vi "test Sort Array of Clusters Natural String Sort.vi"(8 "error in (no error)":errorcluster, 11 "TestCase in":refnum<class "UI Common Unit Tests.lvclass">) -> (0 "error out":errorcluster, 3 "TestCase out":refnum<class "UI Common Unit Tests.lvclass">)   [LabVIEW 2017, in "UI Common Unit Tests.lvclass"]
uses:
  UI Common Unit Tests.lvclass
  Array Row.ctl
  63dc8703-c824-4b80-a085-58f57073aca5.vi
  d8dc5a30-59fd-40f1-b092-92b0634dc405.vi
  c62d43f3-ccf2-448e-89d3-d67a32af4b30.vi
  0d07b81e-88f3-4258-8836-385d3b76f707.vi
  63dc8703-c824-4b80-a085-58f57073aca5.vi/7dda6a87-888e-4219-9294-afb2d8f7f202.vi
  63dc8703-c824-4b80-a085-58f57073aca5.vi/7a811afe-08d6-4889-9a6b-707c54def933.vi
  d8dc5a30-59fd-40f1-b092-92b0634dc405.vi/55d2f0e8-b25a-4c34-86b0-45c4342d676d.vi
  d8dc5a30-59fd-40f1-b092-92b0634dc405.vi/529c5265-cbd4-4584-81ba-3b6ee758e69e.vi
  c62d43f3-ccf2-448e-89d3-d67a32af4b30.vi/6e754a95-77fb-4ec3-a969-ba8b3d19ed54.vi
  c62d43f3-ccf2-448e-89d3-d67a32af4b30.vi/98e32075-a747-4c62-ac3b-b709402c5c03.vi
  0d07b81e-88f3-4258-8836-385d3b76f707.vi/cc1b897a-72e7-4acf-8e52-5fbb4102f40d.vi
  0d07b81e-88f3-4258-8836-385d3b76f707.vi/2126984c-6580-428d-86be-ed2c8ec06a10.vi
  Natural String Merge Sort.vi
  <vilib>/addons/_JKI Toolkits/VI Tester/TestCase.llb/TestCase.lvclass
  C:/Program Files (x86)/National Instruments/LabVIEW 2017/vi.lib/addons/_JKI Toolkits/VI Tester/TestCase.llb/TestCase.lvclass
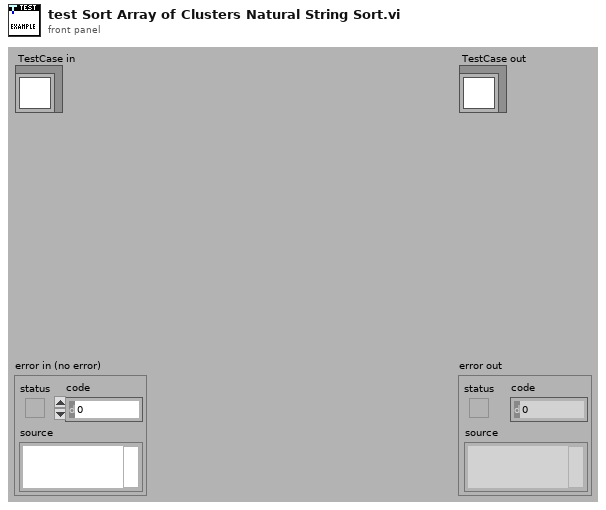
[diagram p1: front panel]
types:
  T1 = typedef "UI Common Unit Tests.lvclass/Array Row.ctl" = cluster{"String":string, "Numeric":dbl}
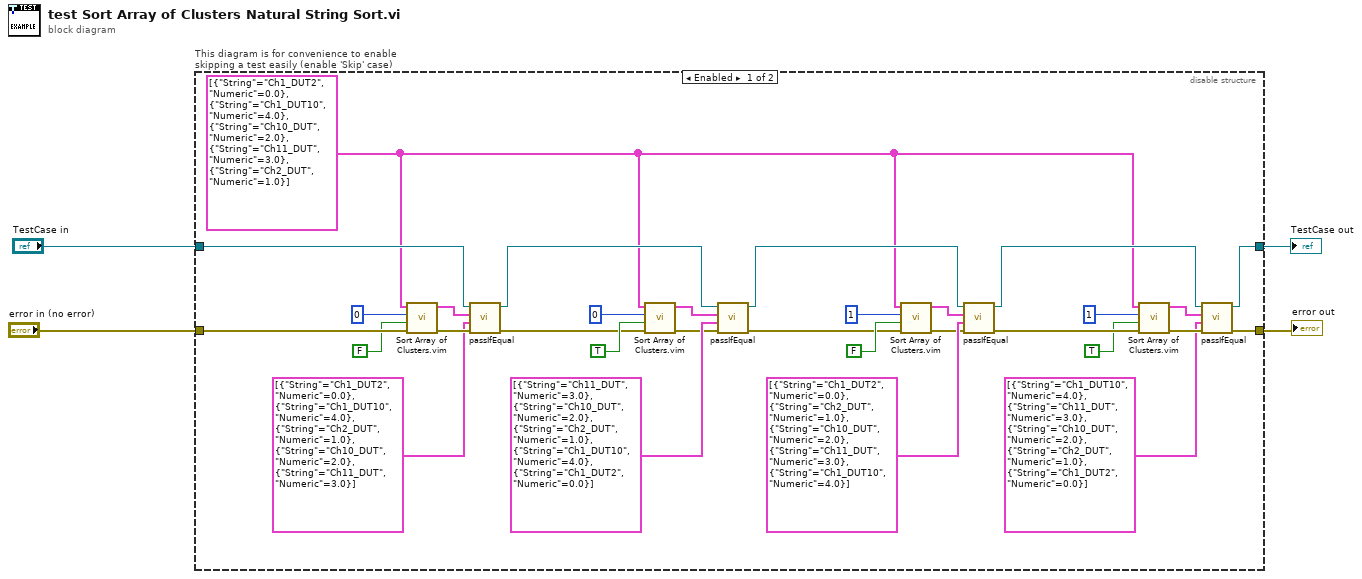
[diagram p0: block diagram]
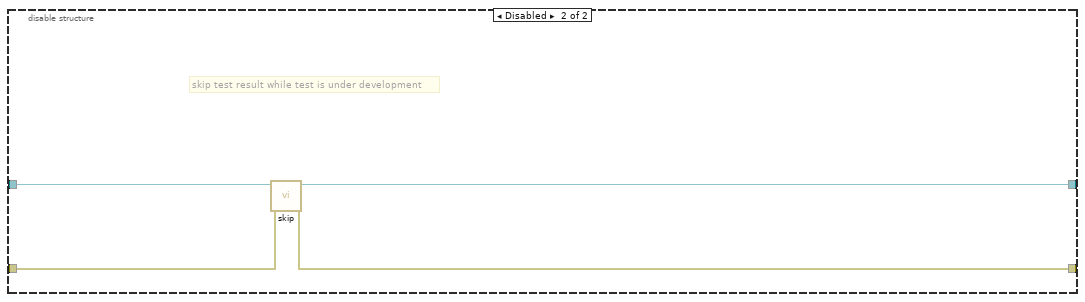
[diagram p2: hidden frame]
diagram:
  n1 = disable-structure "This diagram is for convenience to enable skipping a test easily (enable 'Skip' case)" shown="Enabled" {
    disable-tunnel: "TestCase in" -> [w31 w39]
    disable-tunnel: [w10 w37] -> w1
    disable-tunnel: [w6 w38] -> w3
    disable-tunnel: "error in (no error)" -> [w35 w36]
    frame Enabled {
      w5 = T1[] [{"String"="Ch1_DUT2", "Numeric"=0.0}, {"String"="Ch1_DUT10", "Numeric"=4.0}, {"String"="Ch10_DUT", "Numeric"=2.0}, {"String"="Ch11_DUT", "Numeric"=3.0}, {"String"="Ch2_DUT", "Numeric"=1.0}] ("Value")
      n2 = call "Sort Array of Clusters.vim"("error in (no error)"=w35, "Descending"=FALSE, "index"=u32 0, "Array"=w5) -> ("error out"=w32:errorcluster, "Sorted Array"=w30:T1[])  [unwired: 6 in]
      n3 = call-dynamic "passIfEqual.vi"("error in (no error)"=w32, "y"=T1[] [{"String"="Ch1_DUT2", "Numeric"=0.0}, {"String"="Ch1_DUT10", "Numeric"=4.0}, {"String"="Ch2_DUT", "Numeric"=1.0}, {"String"="Ch10_DUT", "Numeric"=2.0}, {"String"="Ch11_DUT", "Numeric"=3.0}] ("Value"), "x"=w30, "TestCase in"=w31) -> ("error out"=w23:errorcluster, "TestCase out"=w22:refnum<class "UI Common Unit Tests.lvclass">)  [unwired: 6 in]
      n4 = call "Sort Array of Clusters.vim"("error in (no error)"=w23, "Descending"=TRUE, "index"=u32 0, "Array"=w5) -> ("error out"=w26:errorcluster, "Sorted Array"=w27:T1[])  [unwired: 6 in]
      n5 = call-dynamic "passIfEqual.vi"("error in (no error)"=w26, "y"=T1[] [{"String"="Ch11_DUT", "Numeric"=3.0}, {"String"="Ch10_DUT", "Numeric"=2.0}, {"String"="Ch2_DUT", "Numeric"=1.0}, {"String"="Ch1_DUT10", "Numeric"=4.0}, {"String"="Ch1_DUT2", "Numeric"=0.0}] ("Value"), "x"=w27, "TestCase in"=w22) -> ("error out"=w7:errorcluster, "TestCase out"=w8:refnum<class "UI Common Unit Tests.lvclass">)  [unwired: 6 in]
      n6 = call "Sort Array of Clusters.vim"("error in (no error)"=w7, "Descending"=FALSE, "index"=u32 1, "Array"=w5) -> ("error out"=w13:errorcluster, "Sorted Array"=w14:T1[])  [unwired: 6 in]
      n7 = call-dynamic "passIfEqual.vi"("error in (no error)"=w13, "y"=T1[] [{"String"="Ch1_DUT2", "Numeric"=0.0}, {"String"="Ch2_DUT", "Numeric"=1.0}, {"String"="Ch10_DUT", "Numeric"=2.0}, {"String"="Ch11_DUT", "Numeric"=3.0}, {"String"="Ch1_DUT10", "Numeric"=4.0}] ("Value"), "x"=w14, "TestCase in"=w8) -> ("error out"=w21:errorcluster, "TestCase out"=w9:refnum<class "UI Common Unit Tests.lvclass">)  [unwired: 6 in]
      n8 = call "Sort Array of Clusters.vim"("error in (no error)"=w21, "Descending"=TRUE, "index"=u32 1, "Array"=w5) -> ("error out"=w18:errorcluster, "Sorted Array"=w17:T1[])  [unwired: 6 in]
      n9 = call-dynamic "passIfEqual.vi"("error in (no error)"=w18, "y"=T1[] [{"String"="Ch1_DUT10", "Numeric"=4.0}, {"String"="Ch11_DUT", "Numeric"=3.0}, {"String"="Ch10_DUT", "Numeric"=2.0}, {"String"="Ch2_DUT", "Numeric"=1.0}, {"String"="Ch1_DUT2", "Numeric"=0.0}] ("Value"), "x"=w17, "TestCase in"=w9) -> ("error out"=w6:errorcluster, "TestCase out"=w10:refnum<class "UI Common Unit Tests.lvclass">)  [unwired: 6 in]
    }
    frame Disabled {
      # "skip test result while test is under development"
      n10 = call <vilib>:"skip.vi"("error in (no error)"=w36, "TestCase in"=w39) -> ("error out"=w38:errorcluster, "TestCase out"=w37:refnum<class "UI Common Unit Tests.lvclass">)  [unwired: 8 in]
    }
  }
  "error out" <- w3
  "TestCase out" <- w1
